vi "Laser Measurement Tool.vi"() -> ()   [LabVIEW 2017]
uses:
  Subsystems/Measurement/Typedefs/Measurement.Type--Enum.ctl
  Subsystems/Measurement/Typedefs/Configuration.SMU--Cluster.ctl
  Subsystems/SMU/Typedefs/Configuration--Cluster.ctl
  Subsystems/Measurement/Typedefs/Configuration.LIA--Cluster.ctl
  Subsystems/LIA/Typedefs/Configuration--Cluster.ctl
  Subsystems/Measurement/Typedefs/Configuration.OPM--Cluster.ctl
  Subsystems/OPM/Typedefs/Configuration--Cluster.ctl
  Subsystems/Measurement/Typedefs/Configuration.OPA--Cluster.ctl
  Subsystems/OPA/Typedefs/Configuration--Cluster.ctl
  Subsystems/Measurement.WavelengthSweeping/Typedefs/Configuration.Measurement--Cluster.ctl
  Subsystems/Measurement.Free/Measurement.Free.lvclass
  D:/upwork/Laser Measurement Tool/Laser/project/Subsystems/Measurement/Measurement.lvclass
  Subsystems/Measurement.Free.UI/Measurement.Free.UI.lvclass
  D:/upwork/Laser Measurement Tool/Laser/project/Subsystems/Measurement.UI/Measurement.UI.lvclass
  Subsystems/Measurement.WavelengthSweeping/Measurement.WavelengthSweeping.lvclass
  Subsystems/Measurement.WavelengthSweeping.UI/Measurement.WavelengthSweeping.UI.lvclass
  Subsystems/Measurement.Free/Typedefs/Configuration--Cluster.ctl
  Subsystems/Measurement.Free/Typedefs/Configuration.Hardware--Cluster.ctl
  Subsystems/Measurement.WavelengthSweeping/Typedefs/Configuration--Cluster.ctl
  Subsystems/Measurement.WavelengthSweeping/Typedefs/Configuration.Hardware--Cluster.ctl
  Subsystems/Measurement/Measurement.lvclass
  Subsystems/OPA.OrpheusHP/OPA.OrpheusHP.lvclass
  Subsystems/OPM.ThorlabsPM400/OPM.ThorlabsPM400.lvclass
  Subsystems/SMU/SMU.lvclass
  Subsystems/OPA/OPA.lvclass
  Subsystems/OPM/OPM.lvclass
  Subsystems/LIA/LIA.lvclass
panel:
  in  "OK":bool
  out "Measurements Tree":string(tree) caption="Chart A"
  in  "Add":bool
  in  "Remove":bool
  in  "Stop":bool
  in  "Start":bool
  in  "Measurement Parameters":T1(tab)
  in  "Delay time, ms":u16=500 step=100
  in  "Accumulation":u16=5 step=1
  in  "Integration time, s":dbl=5.0 step=0.1
  in  "OPA number of points":u16 step=1
  in  "OPA scan resolution, nm":dbl=20.0 step=10.0 format="%#_6f"
  in  "OPA stop wavelength, nm":dbl=1000.0 step=20.0 format="%#_6f"
  in  "OPA start wavelength, nm":dbl=600.0 step=20.0 format="%#_6f"
  in  "SMU voltage, V":dbl=1.0 step=0.01 format="%#_6f"
  in  "Sync":bool
  in  "Save":bool
  in  "Hardware Parameters":enum32{"Free"}(tab)
  in  "OPA Refresh List":bool
  in  "OPA Serial Number":string(combo)
  in  "OPM Refresh List":bool
  in  "OPM Simulated":bool
  in  "OPM Resource Name":string(combo)
  in  "SMU Channel":string(combo)="A"
  in  "SMU Simulated":bool
  in  "SMU VISA Resource Name":refnum<visa-resource-name>="GPIB0::26::INSTR"
  in  "LIA Simulated":bool
  in  "LIA VISA Resource Name":refnum<visa-resource-name>="GPIB0::8::INSTR"
  in  "Close":bool
  out "Status":string
  out "Progress":u8(slide) scale=0.0..100.0
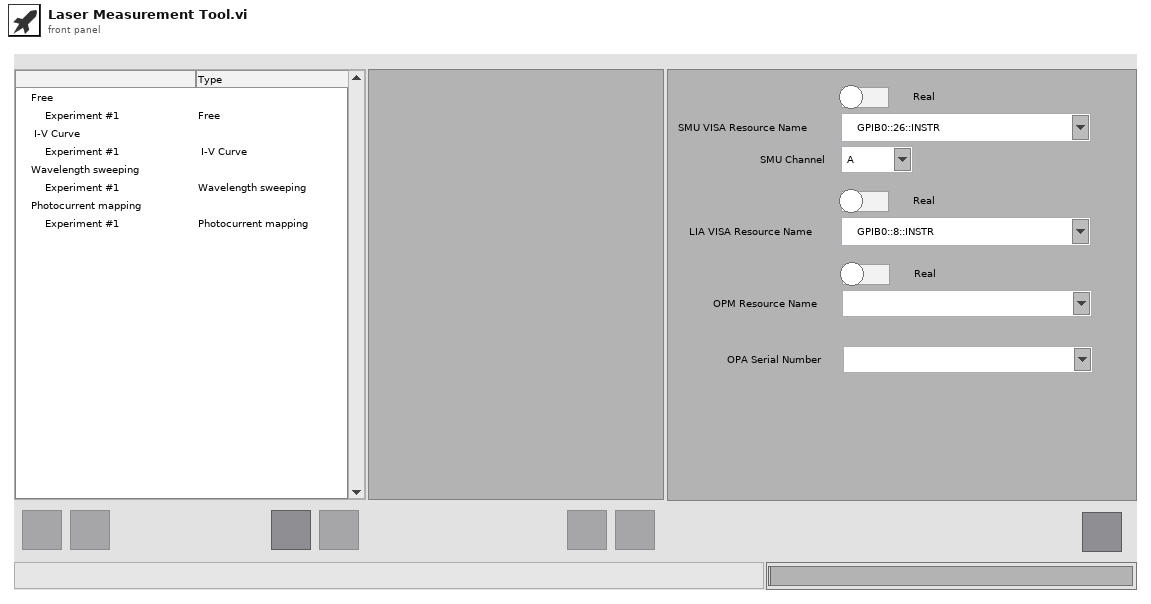
[diagram p1: front panel]
types:
  T1 = enum32{"Free", "I-V Curve", "Wavelength Sweeping", "Photocurrent mapping"}
  T2 = enum8{"Enabled", "Disabled", "Disabled and Grayed Out"}
  T3 = enum32{"Invalid", "Standard", "Closed", "Hidden", "Minimized", "Maximized"}
  T4 = enum32{"invalid app kind", "Development System", "Run Time System", "Student Edition", "Embedded LabVIEW", "Evaluation", "Custom"}
  T5 = typedef "Measurement.lvclass/Measurement.Type--Enum.ctl" = enum16{"Free", "I/V Curve", "Wavelength sweeping", "Photocurrent mapping"}
  T6 = typedef "LVPoint32TypeDef.ctl" = cluster{"Horizontal":i32, "Vertical":i32}
  T7 = typedef "Measurement.lvclass/Configuration.SMU--Cluster.ctl" = cluster{"Enable":bool, "SMU Model":string, "Configuration":T8}
  T8 = typedef "SMU.lvclass/Configuration--Cluster.ctl" = cluster{"VISA Resource":string, "Channel":string}
  T9 = typedef "Measurement.lvclass/Configuration.LIA--Cluster.ctl" = cluster{"Enable":bool, "LIA Model":string, "Configuration":T10}
  T10 = typedef "LIA.lvclass/Configuration--Cluster.ctl" = cluster{"VISA Resource":string}
  T11 = typedef "Measurement.lvclass/Configuration.OPM--Cluster.ctl" = cluster{"Enable":bool, "OPM Model":string, "Configuration":T12}
  T12 = typedef "OPM.lvclass/Configuration--Cluster.ctl" = cluster{"VISA Resource":string}
  T13 = typedef "Measurement.lvclass/Configuration.OPA--Cluster.ctl" = cluster{"Enable":bool, "OPA Model":string, "Configuration":T14}
  T14 = typedef "OPA.lvclass/Configuration--Cluster.ctl" = cluster{"Serial Number":string}
  T15 = typedef "Measurement.WavelengthSweeping.lvclass/Configuration.Measurement--Cluster.ctl" = cluster{"SMU Voltage, V":dbl, "OPA Start wavelength, nm":dbl, "OPA Stop wavelength, nm":dbl, "OPA Scan resolution, nm":dbl, "OPA Number or points":u16, "Integration time, sec":dbl, "Delay time, ms":u16, "Accumulation":u16}
  T16 = cluster{"Core":cluster{"Current VI Reference":refnum<vi>, "Close Panel on Exit?":bool}, "Measurements Tree":refnum<vi>, "Measurement.Type":T5, "Configuration":variant, "Configuration.SMU":T7, "Configuration.LIA":T9, "Configuration.OPM":T11, "Configuration.OPA":T13, "Configuration.Measurement.W-Sweep":T15}
  T17 = cluster{"Current VI Reference":refnum<vi>, "Close Panel on Exit?":bool}
  T18 = typedef "Measurement.Free.lvclass/Configuration--Cluster.ctl" = cluster{"Measurement.Type":T5, "Hardware":T19}
  T19 = typedef "Measurement.Free.lvclass/Configuration.Hardware--Cluster.ctl" = cluster{"SMU":T7, "LIA":T9, "OPM":T11, "OPA":T13}
  T20 = typedef "Measurement.WavelengthSweeping.lvclass/Configuration--Cluster.ctl" = cluster{"Measurement.Type":T5, "Hardware":T21, "Measurement":T15}
  T21 = typedef "Measurement.WavelengthSweeping.lvclass/Configuration.Hardware--Cluster.ctl" = cluster{"SMU":T7, "LIA":T9, "OPM":T11, "OPA":T13}
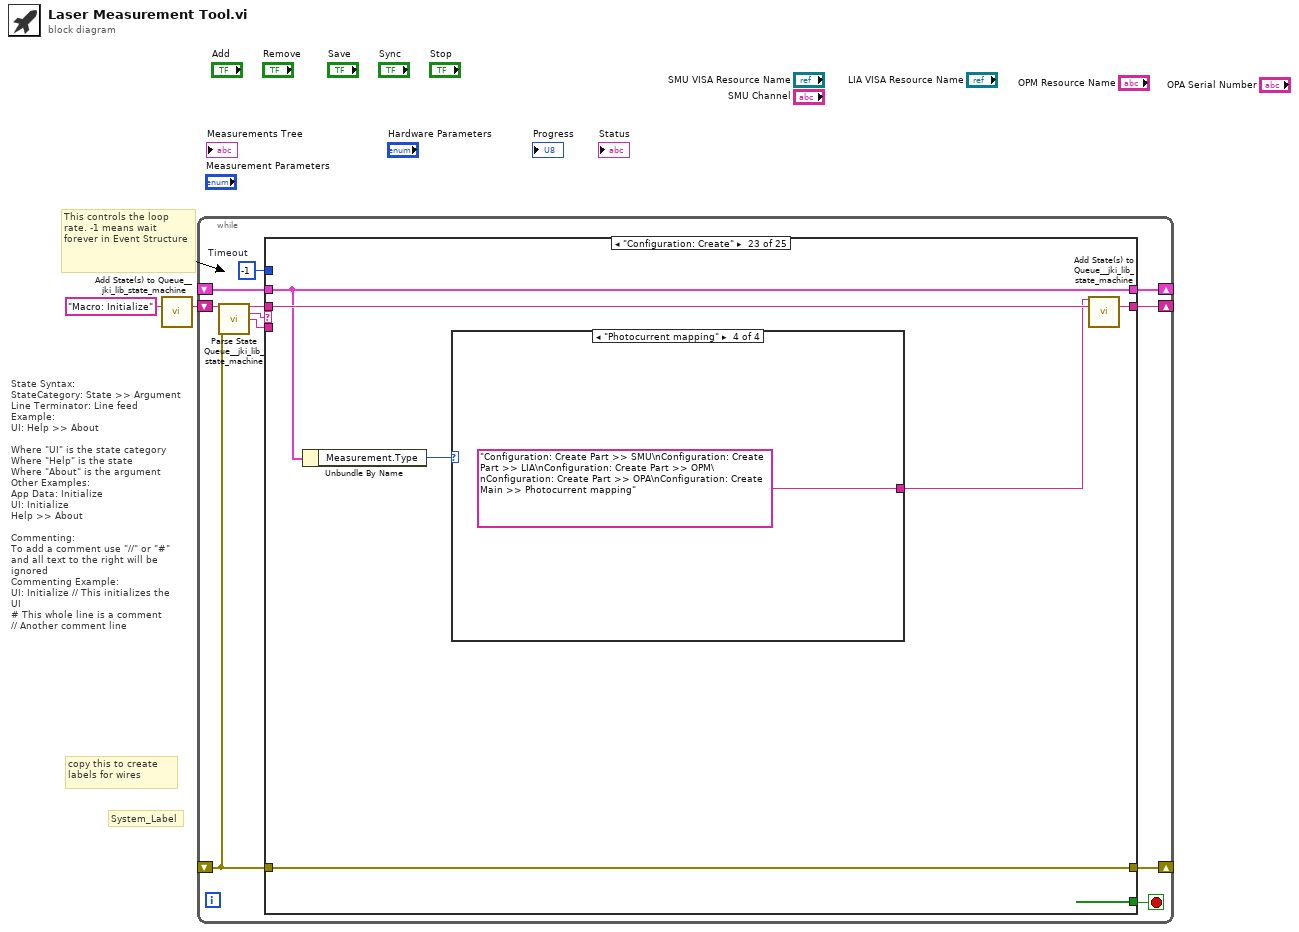
[diagram p0: block diagram]
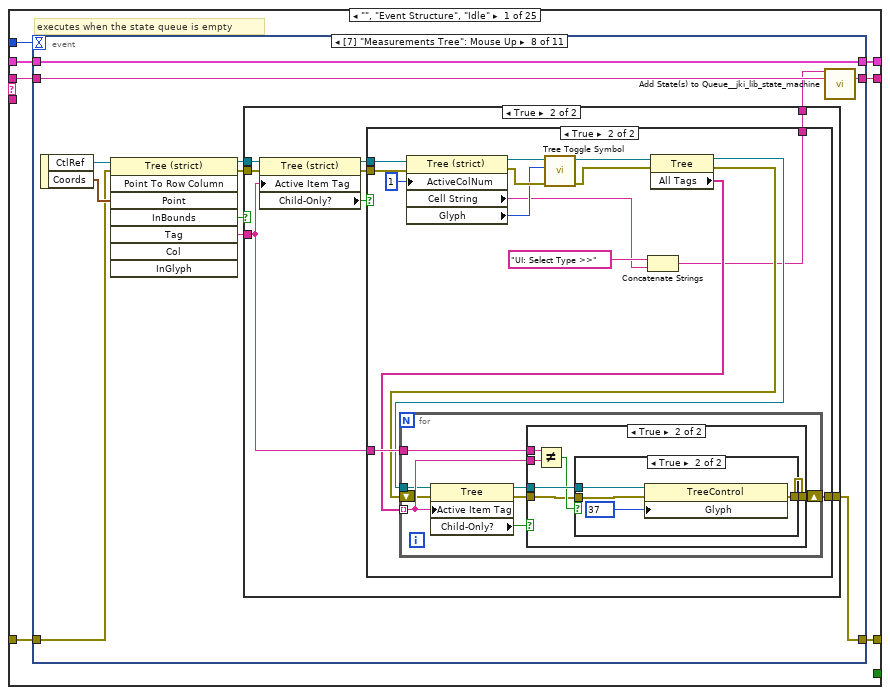
[diagram p2: hidden frame]
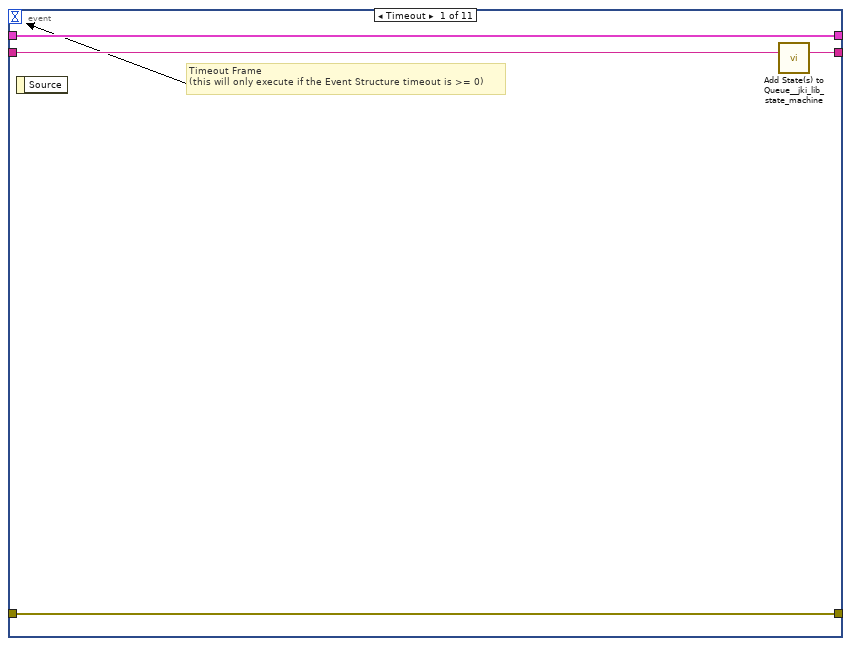
[diagram p3: hidden frame]
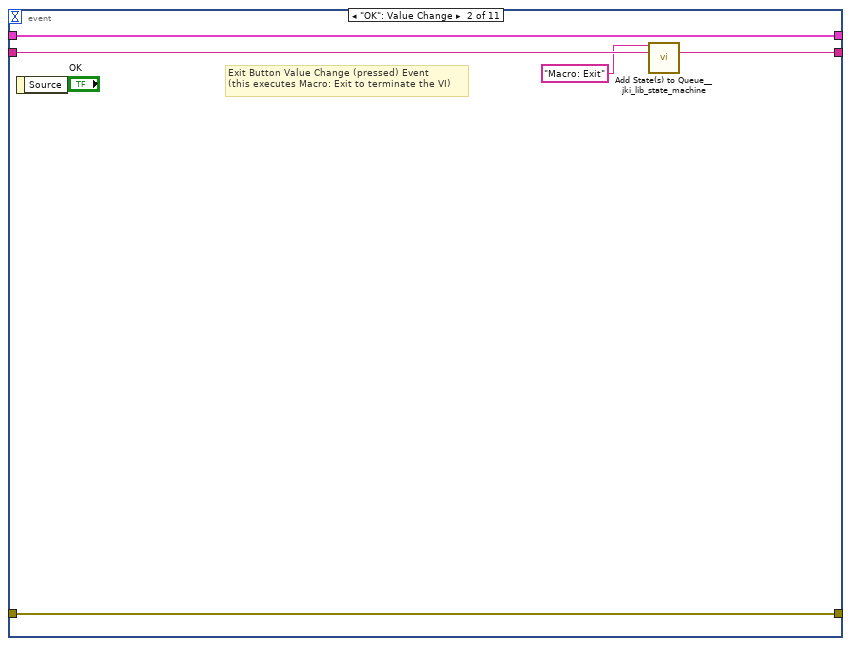
[diagram p4: hidden frame]
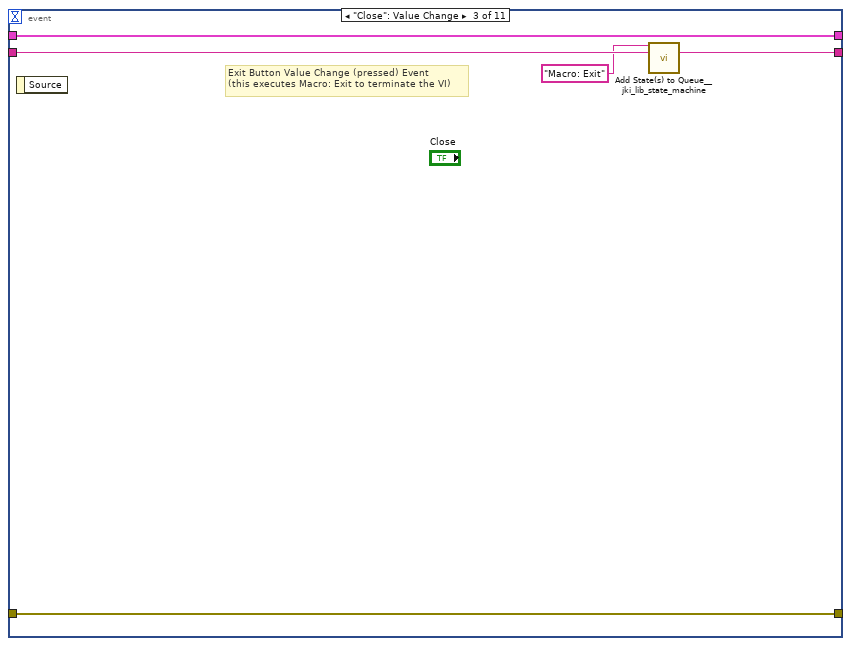
[diagram p5: hidden frame]
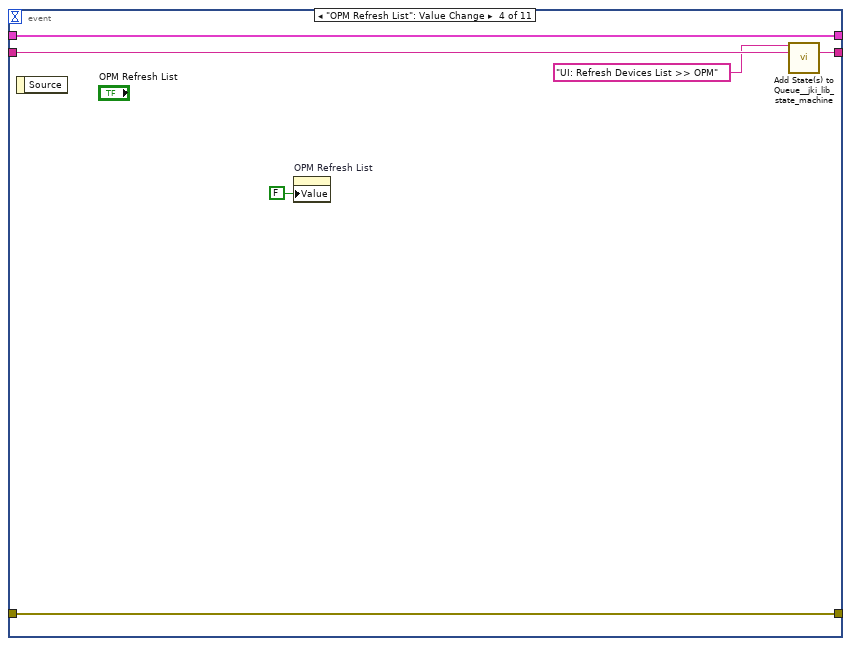
[diagram p6: hidden frame]
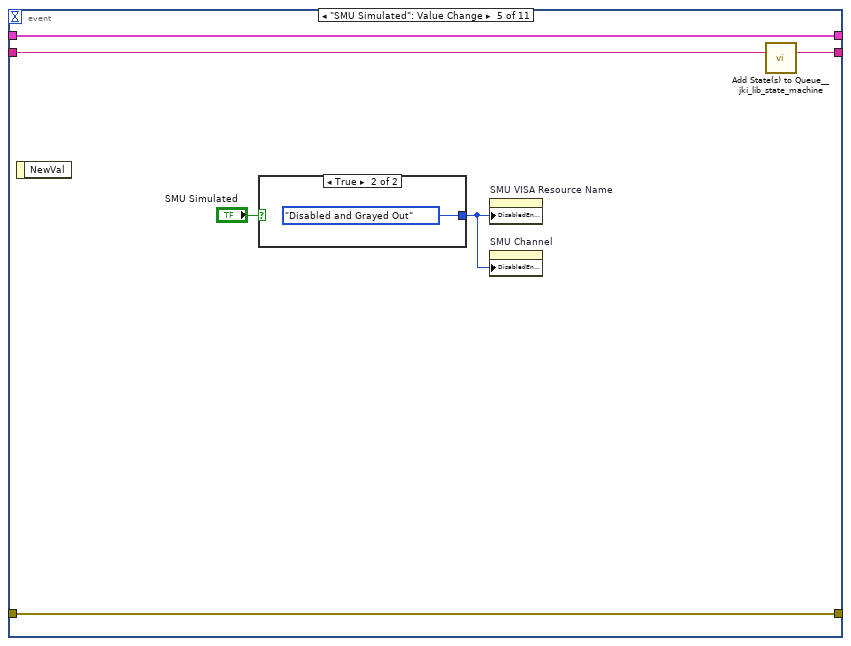
[diagram p7: hidden frame]
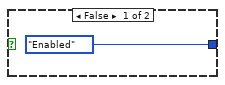
[diagram p8: hidden frame]
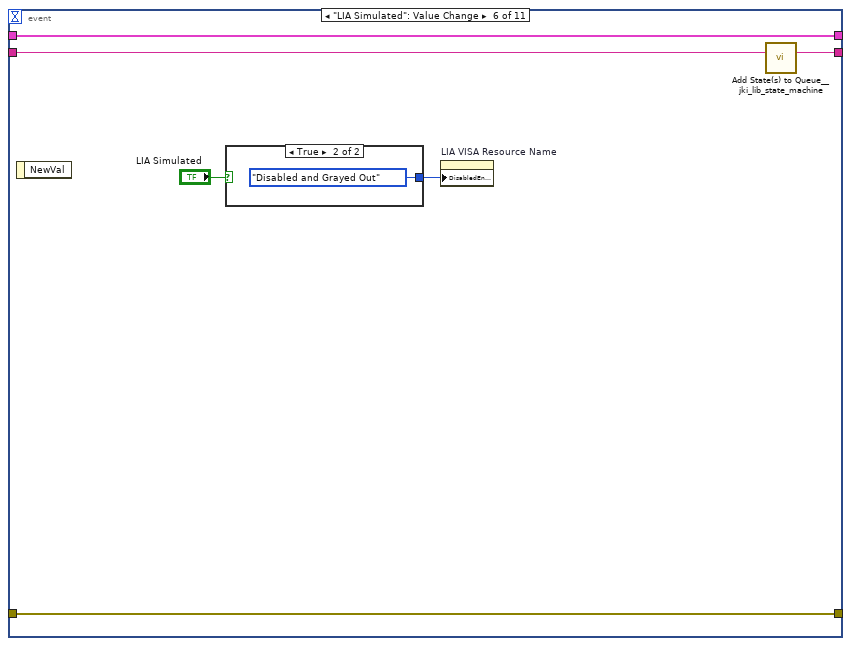
[diagram p9: hidden frame]
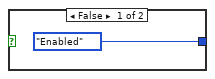
[diagram p10: hidden frame]
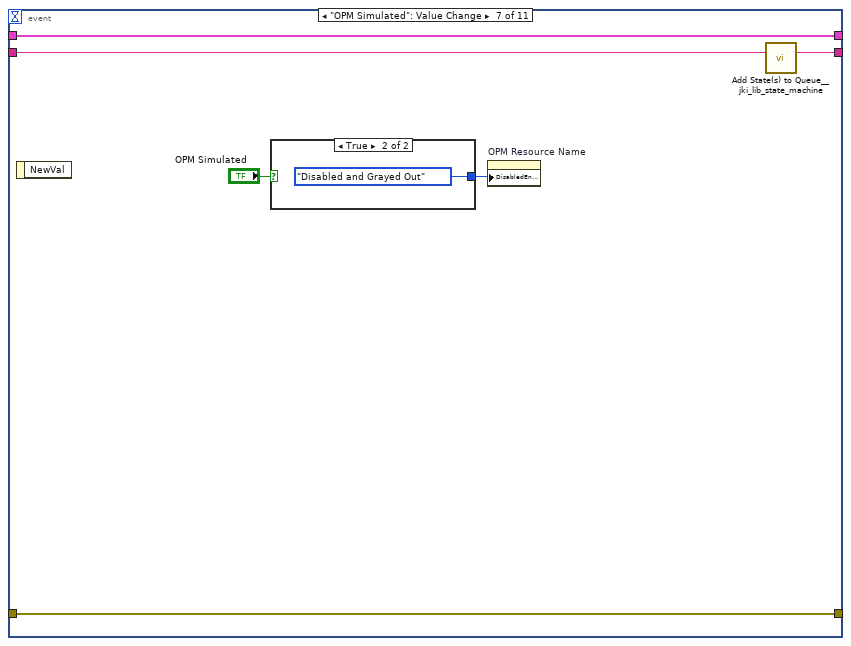
[diagram p11: hidden frame]
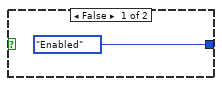
[diagram p12: hidden frame]
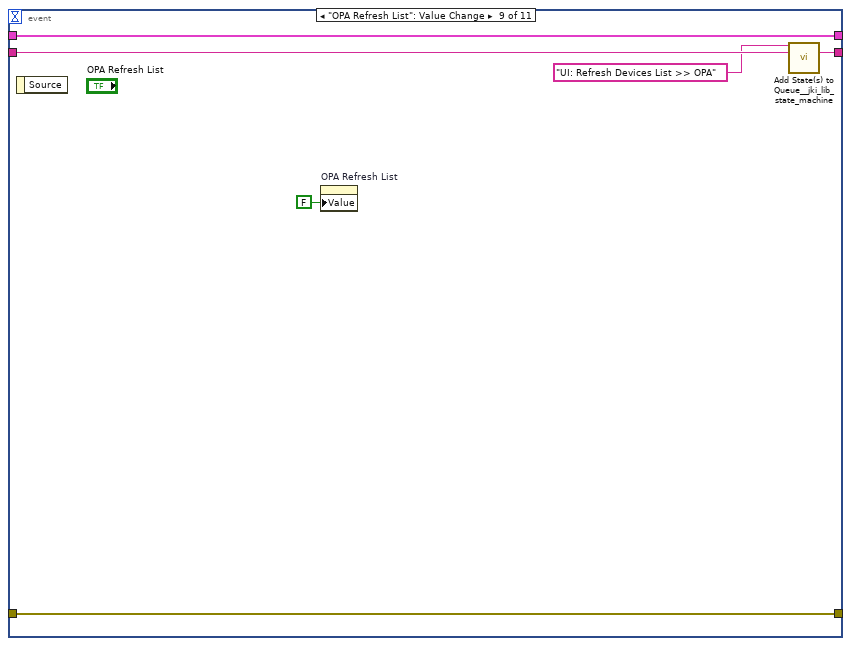
[diagram p17: hidden frame]
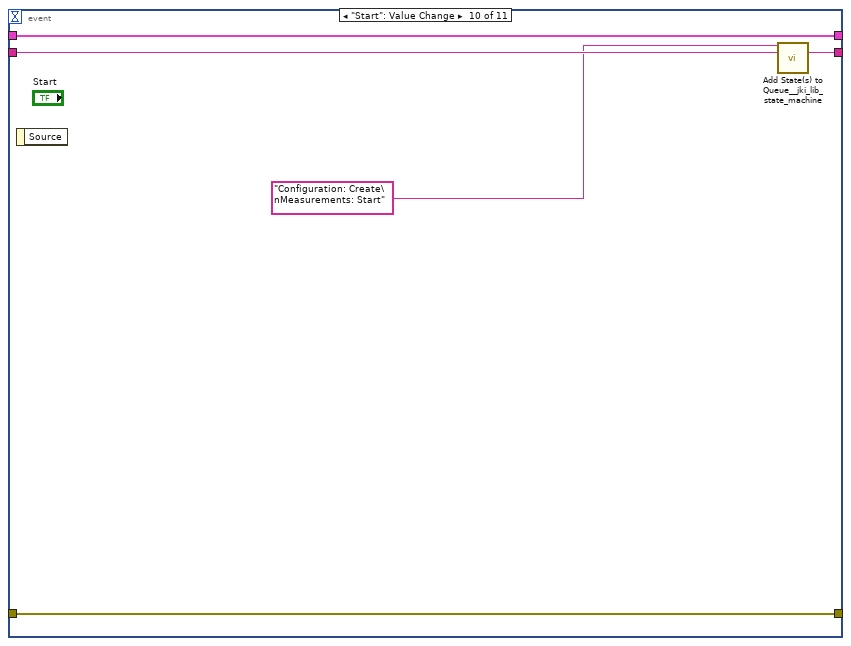
[diagram p18: hidden frame]
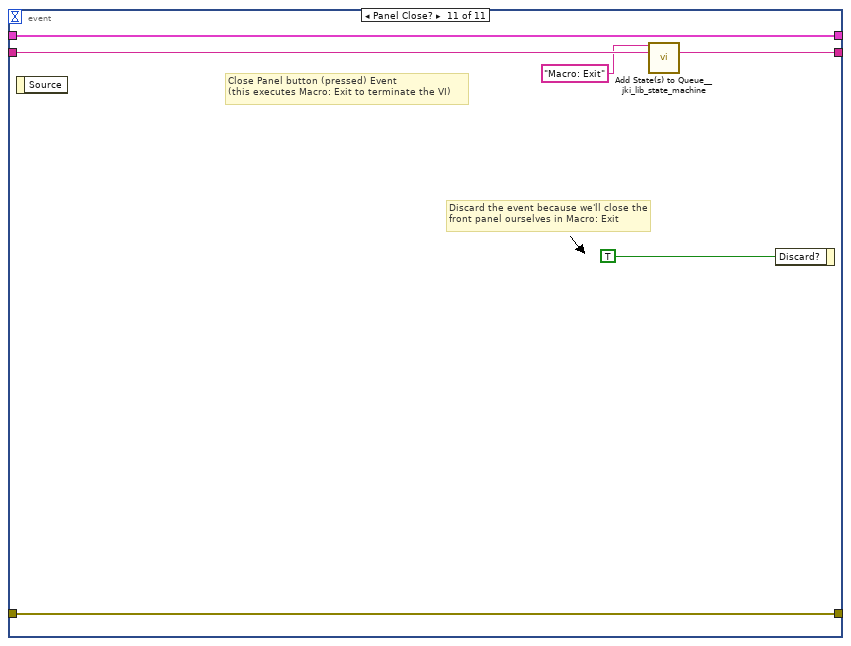
[diagram p19: hidden frame]
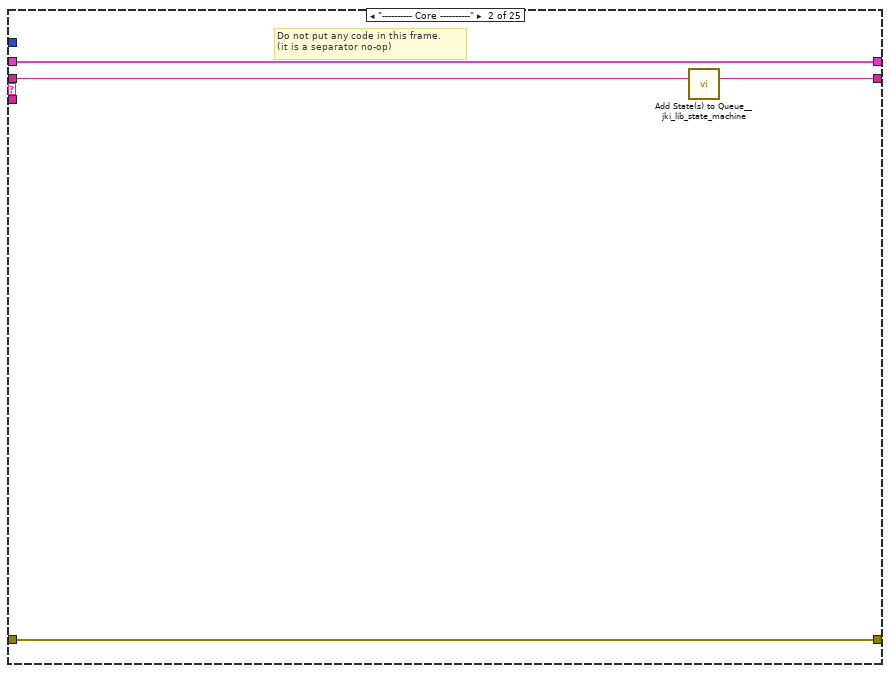
[diagram p20: hidden frame]
diagram:
  # "State Syntax:\nStateCategory: State >> Argument\nLine Terminator: Line feed\nExample:\nUI: Help >> About\n\nWhere \"UI\" is the state category\nWhere \"Help\" is the state\nWhere \"About\" is the argument\nOther Examples:\nApp Data: Initialize\nUI: Initialize\nHelp >> About\n\nCommenting:\nTo add a comment use \"//\" or \"#\" and all text to the right will be ignored\nCommenting Example:\nUI: Initialize // This initializes the UI\n# This whole line is a comment\n// Another comment line"
  # "copy this to create labels for wires"
  # "This controls the loop rate. -1 means wait forever in Event Structure"
  # "System_Label"
  n1 = call <vilib>:"Add State(s) to Queue__jki_lib_state_machine.vi"("State(s) in (\"\")"="Macro: Initialize") -> ("States Out"=w2:string)  [unwired: 14 in]
  n2 = while {
    shift-right: [w6] -> _
    shift-left: _ -> [w5]
    shift-right: [w9] -> _
    shift-left: _ -> [w3]
    shift-right: [w8] -> _
    shift-left: w2 -> [w10]
    stop <- w7 stop-if-true
    w4 = -1  # Timeout
    n3 = call <vilib>:"Parse State Queue__jki_lib_state_machine.vi"("State Queue"=w10, "Error In (no error)"=w3) -> ("Remaining States"=w12:string, "Current State"=w13:string, "Arguments"=w11:string)  [unwired: 11 in]
    n4 = case shown="\"Configuration: Create\"" w13 {
      selector: w13 -> [_ _ w144 _ _ _ _ _ _ _ _ _ _ _ _ _ _ _ _ _ _ _ _ _ _]
      tunnel: w12 -> [w20 w143 w148 w167 w173 w178 w182 w195 w201 w205 w210 w237 w260 w269 w282 w353 w377 w382 w392 w396 w405 w417 w423 w433 w489]
      tunnel: w11 -> [_ _ _ _ _ _ _ _ _ _ _ _ w255 w265 w276 w350 _ _ _ _ _ _ _ w430 w486]
      tunnel: w5 -> [w18 w140 w146 w160 w170 w176 w179 _ w196 w202 w208 w234 w258 w266 w278 w349 w374 w379 w389 w393 w403 w414 w420 w429 w485]
      tunnel: [w17 w141 w150 w164 errorcluster {"status"=FALSE, "code"=0, "source"=""} ("error out") w175 w180 w192 w197 w203 w207 w216 w256 w267 w279 w351 w375 w380 w390 w394 w398 w415 w421 w431 w487] -> w9
      tunnel: w3 -> [w16 w141 w149 w164 w169 w175 w180 w192 w198 w203 w207 w221 w257 w267 w280 w351 w375 w380 w390 w394 w399 w415 w421 w431 w487]
      tunnel: [w19 w142 w147 w166 w172 w177 w181 w194 w200 w204 w209 w236 w259 w268 w281 w352 w376 w381 w391 w395 w404 w416 w422 w432 w488] -> w8
      tunnel: [_ _ _ _ _ TRUE _ _ _ _ _ _ _ _ _ _ _ _ _ _ _ _ _ _ _] -> w7
      tunnel: [w15 w140 w146 w165 w170 w176 w179 w193 w196 w202 w208 w234 w258 w266 w278 w348 w374 w379 w389 w393 w403 w414 w420 w428 w484] -> w6
      tunnel: w4 -> [w14 _ _ _ _ _ _ _ _ _ _ _ _ _ _ _ _ _ _ _ _ _ _ _ _]
      frame "", "Event Structure", "Idle" {
        # "executes when the state queue is empty"
        n5 = event shown="[7] \"Measurements Tree\": Mouse Up" {
          selector: _ -> [_ _ _ _ _ _ _ _ _ _ _]
          dyn-events: _ -> [_ _ _ _ _ _ _ _ _ _ _]
          timeout: w14 -> [_ _ _ _ _ _ _ _ _ _ _]
          tunnel: w20 -> [w24 w29 w34 w40 w42 w52 w60 w74 w128 w131 w139]
          tunnel: [w23 w28 w33 w39 w43 w53 w61 w75 w127 w132 w138] -> w19
          tunnel: w18 -> [w21 w26 w31 w37 w44 w54 w62 w76 w125 w133 w136]
          tunnel: [w22 w27 w32 w38 w41 w51 w59 w67 w126 w130 w137] -> w17
          tunnel: w16 -> [w22 w27 w32 w38 w41 w51 w59 w66 w126 w130 w137]
          tunnel: [w21 w26 w31 w37 w44 w54 w62 w76 w125 w133 w136] -> w15
          event Timeout {
            # "Timeout Frame\n(this will only execute if the Event Structure timeout is >= 0)"
            n6 = event-data() -> ()  [unwired: 1 in, 1 out]
            n7 = call <vilib>:"Add State(s) to Queue__jki_lib_state_machine.vi"("State(s) in (\"\")"=w24) -> ("States Out"=w23:string)  [unwired: 14 in]
          }
          event "OK": Value Change {
            # "Exit Button Value Change (pressed) Event\n(this executes Macro: Exit to terminate the VI)"
            n8 = event-data() -> ()  [unwired: 1 in, 1 out]
            n9 = call <vilib>:"Add State(s) to Queue__jki_lib_state_machine.vi"("State(s) in Front (\"\")"="Macro: Exit", "State(s) in (\"\")"=w29) -> ("States Out"=w28:string)  [unwired: 13 in]
          }
          event "Close": Value Change {
            # "Exit Button Value Change (pressed) Event\n(this executes Macro: Exit to terminate the VI)"
            n10 = event-data() -> ()  [unwired: 1 in, 1 out]
            n11 = call <vilib>:"Add State(s) to Queue__jki_lib_state_machine.vi"("State(s) in Front (\"\")"="Macro: Exit", "State(s) in (\"\")"=w34) -> ("States Out"=w33:string)  [unwired: 13 in]
          }
          event "OPM Refresh List": Value Change {
            n12 = event-data() -> ()  [unwired: 1 in, 1 out]
            n13 = property on="OPM Refresh List" class="Bool (strict)"("Value"=FALSE ("OPM Refresh List")) -> ()  [unwired: 2 in, 2 out]
            n14 = call <vilib>:"Add State(s) to Queue__jki_lib_state_machine.vi"("State(s) in Front (\"\")"="UI: Refresh Devices List >> OPM", "State(s) in (\"\")"=w40) -> ("States Out"=w39:string)  [unwired: 13 in]
          }
          event "SMU Simulated": Value Change {
            n15 = event-data() -> ()  [unwired: 1 in, 1 out]
            n16 = case shown="True" "SMU Simulated" {
              tunnel: [T2."Enabled" ("Disabled") T2."Disabled and Grayed Out" ("Disabled")] -> w46
              frame False {
              }
              frame True {
              }
            }
            n17 = property on="SMU VISA Resource Name" class="VISAName"("DisabledEnum"=w46) -> ()  [unwired: 2 in, 2 out]
            n18 = property on="SMU Channel" class="CmbBox"("DisabledEnum"=w46) -> ()  [unwired: 2 in, 2 out]
            n19 = call <vilib>:"Add State(s) to Queue__jki_lib_state_machine.vi"("State(s) in (\"\")"=w42) -> ("States Out"=w43:string)  [unwired: 14 in]
          }
          event "LIA Simulated": Value Change {
            n20 = event-data() -> ()  [unwired: 1 in, 1 out]
            n21 = case shown="True" "LIA Simulated" {
              tunnel: [T2."Enabled" ("Disabled") T2."Disabled and Grayed Out" ("Disabled")] -> w50
              frame False {
              }
              frame True {
              }
            }
            n22 = property on="LIA VISA Resource Name" class="VISAName"("DisabledEnum"=w50) -> ()  [unwired: 2 in, 2 out]
            n23 = call <vilib>:"Add State(s) to Queue__jki_lib_state_machine.vi"("State(s) in (\"\")"=w52) -> ("States Out"=w53:string)  [unwired: 14 in]
          }
          event "OPM Simulated": Value Change {
            n24 = event-data() -> ()  [unwired: 1 in, 1 out]
            n25 = case shown="True" "OPM Simulated" {
              tunnel: [T2."Enabled" ("Disabled") T2."Disabled and Grayed Out" ("Disabled")] -> w58
              frame False {
              }
              frame True {
              }
            }
            n26 = property on="OPM Resource Name" class="CmbBox"("DisabledEnum"=w58) -> ()  [unwired: 2 in, 2 out]
            n27 = call <vilib>:"Add State(s) to Queue__jki_lib_state_machine.vi"("State(s) in (\"\")"=w60) -> ("States Out"=w61:string)  [unwired: 14 in]
          }
          event "Measurements Tree": Mouse Up {
            n28 = event-data() -> ("CtlRef"=w73:refnum<vi>, "Coords"=w72:T6)  [unwired: 1 in]
            n29 = invoke class="Tree (strict)" method="Point To Row Column"(reference=w73, error in=w66, "Point"=w72) -> (reference out=w70:refnum<vi>, error out=w69:errorcluster, "InBounds"=w71:bool, "Tag"=w68:string)  [unwired: 5 in, 4 out]
            n30 = case shown="True" w71 {
              tunnel: w70 -> [_ w85]
              tunnel: w69 -> [w77 w84]
              tunnel: w68 -> [_ w80]
              tunnel: [w77 w79] -> w67
              tunnel: [_ w78] -> w65
              frame False {
              }
              frame True {
                n31 = property class="Tree (strict)"(reference=w85, error in=w84, "Active Item Tag"=w80) -> (reference out=w82:refnum<vi>, error out=w81:errorcluster, "Child-Only?"=w83:bool)
                n32 = case shown="True" w83 {
                  tunnel: w82 -> [_ w101]
                  tunnel: w81 -> [w86 w102]
                  tunnel: w80 -> [_ w94]
                  tunnel: [w86 w88] -> w79
                  tunnel: [_ w87] -> w78
                  frame False {
                  }
                  frame True {
                    n33 = property class="Tree (strict)"(reference=w101, error in=w102, "ActiveColNum"=1 ("Active Cell:Active Column Number")) -> (reference out=w99:refnum<vi>, error out=w98:errorcluster, "Cell String"=w95:string, "Glyph"=w97:i32)
                    n34 = call "Tree Toggle Symbol.vi"("error in (no error)"=w98, "Symbol"=w97, "TreeControl in"=w99) -> ("error out"=w92:errorcluster, "TreeControl out"=w93:refnum<vi>)  [unwired: 6 in, 1 out]
                    n35 = Concatenate Strings("UI: Select Type >>", w95) -> (w87:string)
                    n36 = property class="Tree"(reference=w93, error in=w92) -> (reference out=w91:refnum<vi>, error out=w90:errorcluster, "All Tags"=w89:string[])
                    n37 = for {
                      tunnel: w89 -> [w108] mode=indexing
                      tunnel: w94 -> [w109]
                      tunnel: w91 -> [w106]
                      shift-right: [w103] -> w88
                      shift-left: w90 -> [w105]
                      n38 = property class="Tree"(reference=w106, error in=w105, "Active Item Tag"=w108) -> (reference out=w107:refnum<vi>, error out=w104:errorcluster, "Child-Only?"=w110:bool)
                      n39 = case shown="True" w110 {
                        tunnel: w109 -> [_ w117]
                        tunnel: w108 -> [_ w116]
                        tunnel: w107 -> [_ w115]
                        tunnel: w104 -> [w111 w113]
                        tunnel: [w111 w112] -> w103
                        frame False {
                        }
                        frame True {
                          n40 = Not Equal?(x=w117, y=w116) -> (x != y?=w114:bool)
                          n41 = case shown="True" w114 {
                            tunnel: w115 -> [_ w122]
                            tunnel: w113 -> [w118 w120]
                            tunnel: [w118 w119] -> w112
                            frame False {
                            }
                            frame True {
                              n42 = property class="TreeControl"(reference=w122, error in=w120, "Glyph"=37) -> (error out=w119:errorcluster)  [unwired: 1 out]
                            }
                          }
                        }
                      }
                    }
                  }
                }
              }
            }
            n43 = call <vilib>:"Add State(s) to Queue__jki_lib_state_machine.vi"("State(s) in Front (\"\")"=w65, "State(s) in (\"\")"=w74) -> ("States Out"=w75:string)  [unwired: 13 in]
          }
          event "OPA Refresh List": Value Change {
            n44 = event-data() -> ()  [unwired: 1 in, 1 out]
            n45 = property on="OPA Refresh List" class="Bool (strict)"("Value"=FALSE ("OPA Refresh List")) -> ()  [unwired: 2 in, 2 out]
            n46 = call <vilib>:"Add State(s) to Queue__jki_lib_state_machine.vi"("State(s) in Front (\"\")"="UI: Refresh Devices List >> OPA", "State(s) in (\"\")"=w128) -> ("States Out"=w127:string)  [unwired: 13 in]
          }
          event "Start": Value Change {
            n47 = event-data() -> ()  [unwired: 1 in, 1 out]
            n48 = call <vilib>:"Add State(s) to Queue__jki_lib_state_machine.vi"("State(s) in Front (\"\")"="Configuration: Create\nMeasurements: Start" ("State(s) in Front (\"\")"), "State(s) in (\"\")"=w131) -> ("States Out"=w132:string)  [unwired: 13 in]
          }
          event Panel Close? {
            # "Discard the event because we'll close the front panel ourselves in Macro: Exit"
            # "Close Panel button (pressed) Event\n(this executes Macro: Exit to terminate the VI)"
            n49 = event-data() -> ()  [unwired: 1 in, 1 out]
            n50 = call <vilib>:"Add State(s) to Queue__jki_lib_state_machine.vi"("State(s) in Front (\"\")"="Macro: Exit", "State(s) in (\"\")"=w139) -> ("States Out"=w138:string)  [unwired: 13 in]
            n51 = event-data("Discard?"=TRUE) -> ()  [unwired: 1 in, 1 out]
          }
        }
      }
      frame "---------- Core ----------" {
        # "Do not put any code in this frame.\n(it is a separator no-op)"
        n52 = call <vilib>:"Add State(s) to Queue__jki_lib_state_machine.vi"("State(s) in (\"\")"=w143) -> ("States Out"=w142:string)  [unwired: 14 in]
      }
      frame Default {
        w153 = 42 items=["No error", "Argument error", "Memory is full", "Out of zone", "End of file", "File already open", "Generic file I/O error", "File not found", "File permission error", "Disk is full", "Duplicate path", "Too many files open", "System feature not enabled", "Resource file not found", "Cannot add resource", "Resource not found", "Image not found", "Image memory error", "Pen does not exist", "Config type invalid", "Config token not found", "Config parse error", "Config memory error", "Bad external code format", "Bad external code offset", "External code not present", "Null window", "Destroy window error", "Null menu", "Print aborted", "Bad print record", "Print driver error", "Windows error during printing", "Memory error during printing", "Print dialog error", "Generic print error", "Invalid device refnum", "Device not found", "Device parameter error", "Device unit error", "Cannot open device", "Device call aborted", "Generic error", "Cancelled by user", "Object ID too low", "Object ID too high", "Object not in heap", "Unknown heap", "Unknown object (invalid DefProc)", "Unknown object (DefProc not in table)", "Message out of range", "Invalid (null) method", "Unknown message", "Manager call not supported", "Bad address", "Network operation in progress", "Network operation timed out", "Connection is busy", "Network attribute not supported", "Network error", "Address in use", "System out of memory", "Connection aborted", "Connection refused", "Not connected", "Already connected", "Connection closed", "Initialization error (interapplication manager)", "Bad occurrence", "Wait on unbound occurrence handler", "Occurrence queue overflow", "Datalog type conflict", "Unused", "Unrecognized type (interapplication manager)", "Memory corrupt", "Failed to make temporary DLL", "Old CIN version", "Drag socket not found", "Failed to load drop-object", "Failed to register OLE object", "Failed to release OLE object", "Format specifier type mismatch", "Unknown format specifier", "Too few format specifiers", "Too many format specifiers", "Scan failed", "Newer CIN version", "Error converting to variant", "Runtime menu error", "Password tampered", "Variant attribute not found", "Incompatible variant data type", "Event data is not available", "Event Store is not present", "Occurrence is not found", "Event Queue is not created", "Event info is not available", "Refnum passed is NULL", "Error retrieving Class GUID", "Error retrieving CoClass GUID", "Error retrieving TypeLib GUID.", "Bad built application magic bytes.", "Specific driver is different from the specific driver associated with the Logical Name.", "There is no session opened to the class driver.", "Max Error", "MAX - Error with config objects", "MAX - Error loading configuration", "MAX - Group not supported"]
        # "Current State"
        # "Do not delete, rename, or modify this frame.\n(this is used to capture unhandled states and typos)"
        # "Handle mistyped state name (developer tool)"
        n53 = Format Into String(format string="Software Exception: Unhandled State \"%s\"." ("message"), error in=w149, w144) -> (resulting string=w152:string, error out=w151:errorcluster)  [unwired: 1 in]
        n54 = call <vilib>:"Error Cluster From Error Code.vi"("show call chain? (False)"=TRUE, "error in (no error)"=w151, "error message (\"\")"=w152, "error code (0)"=w153) -> ("error out"=w150:errorcluster)  [unwired: 5 in]
        n55 = call <vilib>:"Add State(s) to Queue__jki_lib_state_machine.vi"("State(s) in (\"\")"=w148) -> ("States Out"=w147:string)  [unwired: 14 in]
      }
      frame "Initialize Core Data" {
        # "Do not delete, rename, or modify this frame.\n(this is used to determine panel behavior on exit)"
        # "originally closed?"
        # "exe?"
        # "If panel starts closed or is an EXE, then close it when we exit"
        n56 = property class="VI"() -> ("FP.State"=w157:T3)  [unwired: 2 in, 2 out]
        n57 = property class="App"() -> ("App.Kind"=w163:T4)  [unwired: 2 in, 2 out]
        n58 = control-ref of="Current VI Reference"() -> (w158:refnum<vi>)
        n59 = Equal?(x=w157, y=T3."Closed" ("Front Panel Window:State")) -> (x = y?=w155:bool)
        n60 = Equal?(x=w163, y=T4."Run Time System" ("Application:Kind")) -> (x = y?=w161:bool)
        n61 = Or(x=w155, y=w161) -> (x .or. y?=w159:bool)
        n62 = Bundle By Name(cluster=w160, "Core.Current VI Reference"=w158, "Core.Close Panel on Exit?"=w159) -> (w165:T16)
        n63 = call <vilib>:"Add State(s) to Queue__jki_lib_state_machine.vi"("State(s) in (\"\")"=w167) -> ("States Out"=w166:string)  [unwired: 14 in]
      }
      frame "Error Handler" {
        # "Unhandled Error -- Display it"
        # "Handle any errors here.\nYou can also output any states to clean-up after errors occur"
        # "Clear error"
        n64 = call <vilib>:"General Error Handler.vi"("error in (no error)"=w169) -> ()  [unwired: 10 in, 5 out]
        n65 = call <vilib>:"Add State(s) to Queue__jki_lib_state_machine.vi"("State(s) in Front (\"\")"="/* Post Error States", "State(s) in (\"\")"=w173) -> ("States Out"=w172:string)  [unwired: 13 in]
      }
      frame "Exit" {
        # "Do not put any code in this frame.\n(No errors that occur here will be handled.)"
        n66 = call <vilib>:"Add State(s) to Queue__jki_lib_state_machine.vi"("State(s) in (\"\")"=w178) -> ("States Out"=w177:string)  [unwired: 14 in]
      }
      frame "---------- Data ----------" {
        # "Do not put any code in this frame.\n(It is a separator no-op. You can make a copy of this frame to create a new Data frame)"
        n67 = call <vilib>:"Add State(s) to Queue__jki_lib_state_machine.vi"("State(s) in (\"\")"=w182) -> ("States Out"=w181:string)  [unwired: 14 in]
      }
      frame "Data: Initialize" {
        w183 = T15 {"SMU Voltage, V"=0.0, "OPA Start wavelength, nm"=0.0, "OPA Stop wavelength, nm"=0.0, "OPA Scan resolution, nm"=0.0, "OPA Number or points"=0, "Integration time, sec"=0.0, "Delay time, ms"=0, "Accumulation"=0}  # Configuration.Measurement.W-Sweep
        w184 = T13 {"Enable"=FALSE, "OPA Model"="", "Configuration"={"Serial Number"=""}}  # Configuration.OPA
        w185 = T11 {"Enable"=FALSE, "OPM Model"="", "Configuration"={"VISA Resource"=""}}  # Configuration.OPM
        w186 = T9 {"Enable"=FALSE, "LIA Model"="", "Configuration"={"VISA Resource"=""}}  # Configuration.LIA
        w187 = T7 {"Enable"=FALSE, "SMU Model"="", "Configuration"={"VISA Resource"="", "Channel"=""}}  # Configuration.SMU
        w188 = variant  # Configuration
        w189 = Measurement.Type--Enum."Free"  # Measurement.Type
        w191 = T17 {"Current VI Reference"=refnum, "Close Panel on Exit?"=FALSE}  # Core
        # "do not delete - used by framework"
        # "Data names and types of shift register data are defined by this bundle."
        # "Initialize the shift-register data, here.\n(data names are defined by what you wire into the bundle function)"
        n68 = control-ref of="Measurements Tree"() -> (w190:refnum<vi>)
        n69 = Bundle("Core"=w191, "Measurements Tree"=w190, "Measurement.Type"=w189, "Configuration"=w188, "Configuration.SMU"=w187, "Configuration.LIA"=w186, "Configuration.OPM"=w185, "Configuration.OPA"=w184, "Configuration.Measurement.W-Sweep"=w183) -> (w193:T16)  [unwired: 1 in]
        n70 = call <vilib>:"Add State(s) to Queue__jki_lib_state_machine.vi"("State(s) in (\"\")"=w195) -> ("States Out"=w194:string)  [unwired: 14 in]
      }
      frame "Data: Cleanup" {
        # "Cleanup any data and references, here.\n(this is called automatically, by the Macro: Exit)"
        n71 = Unbundle By Name(w196) -> ("Core.Current VI Reference"=w199:refnum<vi>)
        n72 = Close Reference(reference=w199, error in (no error)=w198) -> (error out=w197:errorcluster)
        n73 = call <vilib>:"Add State(s) to Queue__jki_lib_state_machine.vi"("State(s) in (\"\")"=w201) -> ("States Out"=w200:string)  [unwired: 14 in]
      }
      frame "---------- UI ----------" {
        # "Do not put any code in this frame.\n(It is a separator no-op. You can make a copy of this frame to create a new UI frame)"
        n74 = call <vilib>:"Add State(s) to Queue__jki_lib_state_machine.vi"("State(s) in (\"\")"=w205) -> ("States Out"=w204:string)  [unwired: 14 in]
      }
      frame "UI: Initialize" {
        # "Initialize the User Interface, here.\n(this is called automatically, by the Macro: Init)"
        n75 = call <vilib>:"Add State(s) to Queue__jki_lib_state_machine.vi"("State(s) in Front (\"\")"="UI: Tree Init\nUI: Refresh Devices List >> OPM\nUI: Refresh Devices List >> OPA\nUI: Select Type >> Free", "State(s) in (\"\")"=w210) -> ("States Out"=w209:string)  [unwired: 13 in]
      }
      frame "UI: Tree Init" {
        # "...add new measurement here..."
        # "Select Free mode \nas default"
        n76 = Unbundle By Name(w234) -> ("Measurements Tree"=w232:refnum<vi>)
        n77 = call <instrlib>:"Tree Empty.vi"("Tree Reference In"=w232, "error in (no error)"=w221) -> ("Tree Reference Out"=w235:refnum<vi>, "error out"=w230:errorcluster)  [unwired: 15 in, 1 out]
        n78 = call "Tree Create Measurement Item.vi"("error in (no error)"=w230, "New Text Value"="Free", "TreeControl in"=w235) -> ("error out"=w229:errorcluster, "Created Tag"=w218:string, "TreeControl out"=w231:refnum<vi>)  [unwired: 6 in]
        n79 = call "Tree Create Measurement Item.vi"("error in (no error)"=w229, "New Text Value"=" I-V Curve", "TreeControl in"=w231) -> ("error out"=w225:errorcluster, "TreeControl out"=w226:refnum<vi>)  [unwired: 6 in, 1 out]
        n80 = call "Tree Create Measurement Item.vi"("error in (no error)"=w225, "New Text Value"="Wavelength sweeping", "TreeControl in"=w226) -> ("error out"=w214:errorcluster, "TreeControl out"=w215:refnum<vi>)  [unwired: 6 in, 1 out]
        n81 = call "Tree Create Measurement Item.vi"("error in (no error)"=w214, "New Text Value"="Photocurrent mapping", "TreeControl in"=w215) -> ("error out"=w212:errorcluster, "TreeControl out"=w211:refnum<vi>)  [unwired: 6 in, 1 out]
        n82 = property on="Property Node" class="Tree"(reference=w211, error in=w212) -> (reference out=w224:refnum<vi>, error out=w222:errorcluster, "All Tags"=w223:string[])
        n83 = for {
          tunnel: w223 -> [w242] mode=indexing
          tunnel: w224 -> [w245]
          tunnel: [w241] -> w217
          shift-right: [w238] -> w219
          shift-left: w222 -> [w240]
          n84 = property class="Tree"(reference=w245, error in=w240, "Active Item Tag"=w242) -> (reference out=w244:refnum<vi>, error out=w239:errorcluster, "Child-Only?"=w243:bool)
          n85 = case shown="True" w243 {
            tunnel: w244 -> [w247 w252]
            tunnel: w242 -> [_ w251]
            tunnel: [w247 w250] -> w241
            tunnel: w239 -> [w246 w249]
            tunnel: [w246 w248] -> w238
            frame False {
            }
            frame True {
              n86 = property class="Tree"(reference=w252, error in=w249, "Active Item Tag"=w251, "Glyph"=37, "SelColor"=u32 16777216) -> (reference out=w250:refnum<vi>, error out=w248:errorcluster)
            }
          }
        }
        n87 = property class="Tree"(reference=w217, error in=w219, "Active Item Tag"=w218, "Glyph"=38) -> (error out=w216:errorcluster)  [unwired: 1 out]
        n88 = call <vilib>:"Add State(s) to Queue__jki_lib_state_machine.vi"("State(s) in (\"\")"=w237) -> ("States Out"=w236:string)  [unwired: 14 in]
      }
      frame "UI: Cursor Set" {
        # "Argument"
        # "Set and Unset Cursor Busy.\n(Usage: \"UI: Cursor Set >> Busy|Idle\")"
        n89 = case shown="\"Idle\", Default" w255 {
          tunnel: w257 -> [w262 w264]
          tunnel: [w261 w263] -> w256
          frame "Idle", Default {
            n90 = call <vilib>:"Unset Busy.vi"("error in (no error)"=w262) -> ("error out"=w261:errorcluster)  [unwired: 10 in]
          }
          frame "Busy" {
            n91 = call <vilib>:"Set Busy.vi"("error in (no error)"=w264) -> ("error out"=w263:errorcluster)  [unwired: 9 in, 1 out]
          }
        }
        n92 = call <vilib>:"Add State(s) to Queue__jki_lib_state_machine.vi"("State(s) in (\"\")"=w260) -> ("States Out"=w259:string)  [unwired: 14 in]
      }
      frame "UI: Refresh Devices List" {
        n93 = case shown="\"OPA\", Default" w265 {
          frame "OPA", Default {
            n94 = invoke on="OPA Serial Number" class="CmbBox" method="Reinit To Default"() -> (error out=w270:errorcluster)  [unwired: 3 in, 2 out]
            n95 = call "Locate Devices.vi"() -> ("Serial Numbers"=w271:string[])  [unwired: 2 in, 1 out]
            n96 = property on="OPA Serial Number" class="CmbBox"(error in=w270, "Strings[]"=w271) -> ()  [unwired: 1 in, 2 out]
            n97 = Index Array(array=w271) -> (element=w272:string)  [unwired: 1 in]
            n98 = property on="OPA Serial Number" class="CmbBox"("Value"=w272) -> ()  [unwired: 2 in, 2 out]
          }
          frame "OPM" {
            n99 = invoke on="OPM Resource Name" class="CmbBox" method="Reinit To Default"() -> (error out=w273:errorcluster)  [unwired: 3 in, 2 out]
            n100 = call "Find Resources.vi"() -> ("Resource Names"=w274:string[])  [unwired: 2 in, 1 out]
            n101 = property on="OPM Resource Name" class="CmbBox"(error in=w273, "Strings[]"=w274) -> ()  [unwired: 1 in, 2 out]
            n102 = Index Array(array=w274) -> (element=w275:string)  [unwired: 1 in]
            n103 = property on="OPM Resource Name" class="CmbBox"("Value"=w275) -> ()  [unwired: 2 in, 2 out]
          }
        }
        n104 = call <vilib>:"Add State(s) to Queue__jki_lib_state_machine.vi"("State(s) in (\"\")"=w269) -> ("States Out"=w268:string)  [unwired: 14 in]
      }
      frame "UI: Front Panel State" {
        # "Argument"
        # "Set Front Panel Open or Closed\n(Usage: \"UI: Front Panel State >> Open|Close\")"
        n105 = Unbundle By Name(w278) -> ("Core.Current VI Reference"=w277:refnum<vi>)
        n106 = case shown="\"Minimize\", \"Minimized\"" w276 {
          tunnel: w280 -> [w288 w303 w314 w327 w340]
          tunnel: [w290 w304 w316 w329 w342] -> w279
          tunnel: w277 -> [w289 w301 w315 w328 w341]
          frame "Open", "Standard", Default {
            w283 = T3."Standard" ("State")
            n107 = property class="VI"(reference=w289, error in=w288) -> (reference out=w286:refnum<vi>, error out=w287:errorcluster, "FP.State"=w285:T3)
            n108 = Not Equal?(x=w285, y=w283) -> (x != y?=w284:bool)
            n109 = case shown="True" w284 {
              tunnel: [w294 w296] -> w290
              tunnel: w287 -> [w293 w296]
              tunnel: w286 -> [w292 _]
              tunnel: w283 -> [w291 _]
              frame True {
                n110 = invoke class="VI" method="FP.Open"(reference=w292, error in=w293, "Activate"=TRUE, "State"=w291) -> (error out=w294:errorcluster)  [unwired: 1 in, 4 out]
              }
              frame False {
              }
            }
          }
          frame "Close", "Closed" {
            n111 = property class="VI"(reference=w301, error in=w303) -> (reference out=w300:refnum<vi>, error out=w302:errorcluster, "FP.State"=w298:T3)
            n112 = Not Equal?(x=w298, y=T3."Closed" ("Front Panel Window:State")) -> (x != y?=w297:bool)
            n113 = case shown="True" w297 {
              tunnel: [w305 w308] -> w304
              tunnel: w302 -> [w305 w307]
              tunnel: w300 -> [_ w306]
              frame False {
              }
              frame True {
                n114 = invoke class="VI" method="FP.Close"(reference=w306, error in=w307) -> (error out=w308:errorcluster)  [unwired: 1 in, 2 out]
              }
            }
          }
          frame "Hidden", "Hide" {
            w309 = T3."Hidden" ("State")
            n115 = property class="VI"(reference=w315, error in=w314) -> (reference out=w312:refnum<vi>, error out=w313:errorcluster, "FP.State"=w311:T3)
            n116 = Not Equal?(x=w311, y=w309) -> (x != y?=w310:bool)
            n117 = case shown="True" w310 {
              tunnel: [w320 w321] -> w316
              tunnel: w313 -> [w319 w321]
              tunnel: w312 -> [w318 _]
              tunnel: w309 -> [w317 _]
              frame True {
                n118 = invoke class="VI" method="FP.Open"(reference=w318, error in=w319, "State"=w317) -> (error out=w320:errorcluster)  [unwired: 2 in, 4 out]
              }
              frame False {
              }
            }
          }
          frame "Minimize", "Minimized" {
            w322 = T3."Minimized" ("State")
            n119 = property class="VI"(reference=w328, error in=w327) -> (reference out=w325:refnum<vi>, error out=w326:errorcluster, "FP.State"=w324:T3)
            n120 = Not Equal?(x=w324, y=w322) -> (x != y?=w323:bool)
            n121 = case shown="True" w323 {
              tunnel: [w333 w334] -> w329
              tunnel: w326 -> [w332 w334]
              tunnel: w325 -> [w331 _]
              tunnel: w322 -> [w330 _]
              frame True {
                n122 = invoke class="VI" method="FP.Open"(reference=w331, error in=w332, "State"=w330) -> (error out=w333:errorcluster)  [unwired: 2 in, 4 out]
              }
              frame False {
              }
            }
          }
          frame "Maximize", "Maximized" {
            w335 = T3."Maximized" ("State")
            n123 = property class="VI"(reference=w341, error in=w340) -> (reference out=w338:refnum<vi>, error out=w339:errorcluster, "FP.State"=w337:T3)
            n124 = Not Equal?(x=w337, y=w335) -> (x != y?=w336:bool)
            n125 = case shown="True" w336 {
              tunnel: [w346 w347] -> w342
              tunnel: w339 -> [w345 w347]
              tunnel: w338 -> [w344 _]
              tunnel: w335 -> [w343 _]
              frame True {
                n126 = invoke class="VI" method="FP.Open"(reference=w344, error in=w345, "State"=w343) -> (error out=w346:errorcluster)  [unwired: 2 in, 4 out]
              }
              frame False {
              }
            }
          }
        }
        n127 = call <vilib>:"Add State(s) to Queue__jki_lib_state_machine.vi"("State(s) in (\"\")"=w282) -> ("States Out"=w281:string)  [unwired: 14 in]
      }
      frame "UI: Select Type" {
        n128 = case shown="\"Free\", Default" w350 {
          tunnel: w349 -> [w358 w363 w366 w373]
          tunnel: [w356 w362 w367 w372] -> w348
          frame "Free", Default {
            n129 = Bundle By Name(cluster=w358, "Measurement.Type"=Measurement.Type--Enum."Free") -> (w356:T16)
            n130 = property on="Measurement Parameters" class="TabCtl (strict)"("Value"=T1."Free" ("Measurement Parameters")) -> ()  [unwired: 2 in, 2 out]
            n131 = property on="Status" class="Str"("Value"="Free measurement mode" ("Status")) -> ()  [unwired: 2 in, 2 out]
          }
          frame "I-V Curve" {
            n132 = Bundle By Name(cluster=w363, "Measurement.Type"=Measurement.Type--Enum."I/V Curve") -> (w362:T16)
            n133 = property on="Measurement Parameters" class="TabCtl (strict)"("Value"=T1."I-V Curve" ("Measurement Parameters")) -> ()  [unwired: 2 in, 2 out]
            n134 = property on="Status" class="Str"("Value"="I/V curve measurement mode" ("Status")) -> ()  [unwired: 2 in, 2 out]
          }
          frame "Wavelength sweeping" {
            n135 = Bundle By Name(cluster=w366, "Measurement.Type"=Measurement.Type--Enum."Wavelength sweeping") -> (w367:T16)
            n136 = property on="Measurement Parameters" class="TabCtl (strict)"("Value"=T1."Wavelength Sweeping" ("Measurement Parameters")) -> ()  [unwired: 2 in, 2 out]
            n137 = property on="Status" class="Str"("Value"=" Wavelength Sweeping measurement mode" ("Status")) -> ()  [unwired: 2 in, 2 out]
          }
          frame "Photocurrent mapping" {
            n138 = Bundle By Name(cluster=w373, "Measurement.Type"=Measurement.Type--Enum."Photocurrent mapping") -> (w372:T16)
            n139 = property on="Measurement Parameters" class="TabCtl (strict)"("Value"=T1."Photocurrent mapping" ("Measurement Parameters")) -> ()  [unwired: 2 in, 2 out]
            n140 = property on="Status" class="Str"("Value"=" Photocurrent mapping measurement mode" ("Status")) -> ()  [unwired: 2 in, 2 out]
          }
        }
        n141 = call <vilib>:"Add State(s) to Queue__jki_lib_state_machine.vi"("State(s) in (\"\")"=w353) -> ("States Out"=w352:string)  [unwired: 14 in]
      }
      frame "---------- Macro ----------" {
        # "Do not put any code in this frame.\n(It is a separator no-op. You can make a copy of this frame to create a new Macro frame)"
        n142 = call <vilib>:"Add State(s) to Queue__jki_lib_state_machine.vi"("State(s) in (\"\")"=w377) -> ("States Out"=w376:string)  [unwired: 14 in]
      }
      frame "Macro: Initialize" {
        # "Initialization Macro\n(This is called once, when the VI starts)"
        n143 = call <vilib>:"Add State(s) to Queue__jki_lib_state_machine.vi"("State(s) in Front (\"\")"="Data: Initialize\nInitialize Core Data\nUI: Initialize\nUI: Front Panel State >> Open", "State(s) in (\"\")"=w382) -> ("States Out"=w381:string)  [unwired: 13 in]
      }
      frame "Macro: Exit" {
        # "Exit Macro\n(This is called once, when the VI exits)"
        n144 = Unbundle By Name(w389) -> ("Core.Close Panel on Exit?"=w388:bool)
        n145 = Select(t="UI: Front Panel State >> Close", s=w388, f="") -> (s? t:f=w385:string)
        n146 = call <vilib>:"Add State(s) to Queue__jki_lib_state_machine.vi"("State(s) in (\"\")"=w385, "State(s) at Back (\"\")"="Data: Cleanup\nExit") -> ("States Out"=w383:string)  [unwired: 13 in]
        n147 = call <vilib>:"Add State(s) to Queue__jki_lib_state_machine.vi"("State(s) in Front (\"\")"=w383, "State(s) in (\"\")"=w392) -> ("States Out"=w391:string)  [unwired: 13 in]
      }
      frame "---------- Measurements ----------" {
        # "Template Separator\n(You can make a copy of, or modify, this frame)"
        n148 = call <vilib>:"Add State(s) to Queue__jki_lib_state_machine.vi"("State(s) in (\"\")"=w396) -> ("States Out"=w395:string)  [unwired: 14 in]
      }
      frame "Measurements: Start" {
        n149 = Unbundle By Name(w403) -> ("Measurement.Type"=w402:T5, "Configuration"=w397:variant)
        n150 = case shown="\"Free\", Default" w402 {
          tunnel: [w407 w409 w411 w413] -> w401
          tunnel: [w406 w408 w410 w412] -> w400
          frame "Free", Default {
            w406 = refnum<class "Measurement.Free.UI.lvclass"> refnum  # Measurement.Free.UI
            w407 = refnum<class "Measurement.Free.lvclass"> refnum  # Measurement.Free
          }
          frame "I/V Curve" {
            w408 = refnum<class "Measurement.Free.UI.lvclass"> refnum  # Measurement.Free.UI
            w409 = refnum<class "Measurement.Free.lvclass"> refnum  # Measurement.Free
          }
          frame "Wavelength sweeping" {
            w410 = refnum<class "Measurement.WavelengthSweeping.UI.lvclass"> refnum  # Measurement.WavelengthSweeping.UI
            w411 = refnum<class "Measurement.WavelengthSweeping.lvclass"> refnum  # Measurement.WavelengthSweeping
          }
          frame "Photocurrent mapping" {
            w412 = refnum<class "Measurement.Free.UI.lvclass"> refnum  # Measurement.Free.UI
            w413 = refnum<class "Measurement.Free.lvclass"> refnum  # Measurement.Free
          }
        }
        n151 = call "Measurement Launcher.vi"("error in (no error)"=w399, "Configuration"=w397, "Measurement.UI"=w400, "Measurement"=w401) -> ("error out"=w398:errorcluster)  [unwired: 7 in]
        n152 = call <vilib>:"Add State(s) to Queue__jki_lib_state_machine.vi"("State(s) in (\"\")"=w405) -> ("States Out"=w404:string)  [unwired: 14 in]
      }
      frame "---------- Configuration ----------" {
        # "Do not put any code in this frame.\n(it is a separator no-op)"
        n153 = call <vilib>:"Add State(s) to Queue__jki_lib_state_machine.vi"("State(s) in (\"\")"=w417) -> ("States Out"=w416:string)  [unwired: 14 in]
      }
      frame "Configuration: Create" {
        n154 = Unbundle By Name(w420) -> ("Measurement.Type"=w419:T5)
        n155 = case shown="\"Photocurrent mapping\"" w419 {
          tunnel: ["Configuration: Create Part >> SMU\nConfiguration: Create Part >> LIA\nConfiguration: Create Part >> OPM\nConfiguration: Create Part >> OPA\nConfiguration: Create Main >> Free" ("State(s) in Front (\"\")") "Configuration: Create Part >> SMU\nConfiguration: Create Part >> LIA\nConfiguration: Create Part >> OPM\nConfiguration: Create Part >> OPA\nConfiguration: Create Main >> I-V Curve" ("State(s) in Front (\"\")") "Configuration: Create Part >> SMU\nConfiguration: Create Part >> LIA\nConfiguration: Create Part >> OPM\nConfiguration: Create Part >> OPA\nConfiguration: Create Main >> Wavelength sweeping" ("State(s) in Front (\"\")") "Configuration: Create Part >> SMU\nConfiguration: Create Part >> LIA\nConfiguration: Create Part >> OPM\nConfiguration: Create Part >> OPA\nConfiguration: Create Main >> Photocurrent mapping" ("State(s) in Front (\"\")")] -> w418
          frame "Free", Default {
          }
          frame "I/V Curve" {
          }
          frame "Wavelength sweeping" {
          }
          frame "Photocurrent mapping" {
          }
        }
        n156 = call <vilib>:"Add State(s) to Queue__jki_lib_state_machine.vi"("State(s) in Front (\"\")"=w418, "State(s) in (\"\")"=w423) -> ("States Out"=w422:string)  [unwired: 13 in]
      }
      frame "Configuration: Create Part" {
        n157 = case shown="\"SMU\", Default" w430 {
          tunnel: w429 -> [w435 w447 w456 w467 w474]
          tunnel: [w434 w446 w457 w466 w473] -> w428
          frame "SMU", Default {
            w439 = T7 {"Enable"=FALSE, "SMU Model"="", "Configuration"={"VISA Resource"="", "Channel"=""}}  # Configuration.SMU
            n158 = property on="SMU Simulated" class="Bool (strict)"() -> ("Value"=w437:bool)  [unwired: 2 in, 2 out]
            n159 = case shown="False" w437 {
              tunnel: ["Keithley2600" ("SMU Model") "Simulated" ("SMU Model")] -> w438
              frame False {
              }
              frame True {
              }
            }
            n160 = property on="SMU VISA Resource Name" class="VISAName"() -> ("Value"=w441:refnum<visa-resource-name>)  [unwired: 2 in, 2 out]
            n161 = property on="SMU Channel" class="CmbBox"() -> ("Value"=w442:string)  [unwired: 2 in, 2 out]
            n162 = Bundle By Name(cluster=w439, "Enable"=TRUE, "SMU Model"=w438, "Configuration.VISA Resource"=w441, "Configuration.Channel"=w442) -> (w436:T7)
            n163 = Bundle By Name(cluster=w435, "Configuration.SMU"=w436) -> (w434:T16)
          }
          frame "LIA" {
            w449 = T9 {"Enable"=FALSE, "LIA Model"="", "Configuration"={"VISA Resource"=""}}  # Configuration.LIA
            n164 = property on="LIA Simulated" class="Bool (strict)"() -> ("Value"=w452:bool)  [unwired: 2 in, 2 out]
            n165 = case shown="False" w452 {
              tunnel: ["SR810" ("SMU Model") "Simulated" ("SMU Model")] -> w450
              frame False {
              }
              frame True {
              }
            }
            n166 = property on="LIA VISA Resource Name" class="VISAName"() -> ("Value"=w451:refnum<visa-resource-name>)  [unwired: 2 in, 2 out]
            n167 = Bundle By Name(cluster=w449, "Enable"=TRUE, "LIA Model"=w450, "Configuration.VISA Resource"=w451) -> (w445:T9)
            n168 = Bundle By Name(cluster=w447, "Configuration.LIA"=w445) -> (w446:T16)
          }
          frame "OPM" {
            w459 = T11 {"Enable"=FALSE, "OPM Model"="", "Configuration"={"VISA Resource"=""}}  # Configuration.OPM
            n169 = property on="OPM Simulated" class="Bool (strict)"() -> ("Value"=w462:bool)  [unwired: 2 in, 2 out]
            n170 = case shown="False" w462 {
              tunnel: ["ThorlabsPM400" ("SMU Model") "Simulated" ("SMU Model")] -> w460
              frame False {
              }
              frame True {
              }
            }
            n171 = property on="OPM Resource Name" class="CmbBox"() -> ("Value"=w461:string)  [unwired: 2 in, 2 out]
            n172 = Bundle By Name(cluster=w459, "Enable"=TRUE, "OPM Model"=w460, "Configuration.VISA Resource"=w461) -> (w455:T11)
            n173 = Bundle By Name(cluster=w456, "Configuration.OPM"=w455) -> (w457:T16)
          }
          frame "OPA" {
            w470 = T13 {"Enable"=FALSE, "OPA Model"="", "Configuration"={"Serial Number"=""}}  # Configuration.OPA
            n174 = property on="OPA Serial Number" class="CmbBox"() -> ("Value"=w471:string)  [unwired: 2 in, 2 out]
            n175 = Bundle By Name(cluster=w470, "Enable"=TRUE, "OPA Model"="OrpheusHP", "Configuration.Serial Number"=w471) -> (w465:T13)
            n176 = Bundle By Name(cluster=w467, "Configuration.OPA"=w465) -> (w466:T16)
          }
          frame "Wavelength sweeping" {
            w475 = T15 {"SMU Voltage, V"=0.0, "OPA Start wavelength, nm"=0.0, "OPA Stop wavelength, nm"=0.0, "OPA Scan resolution, nm"=0.0, "OPA Number or points"=0, "Integration time, sec"=0.0, "Delay time, ms"=0, "Accumulation"=0}  # Configuration.Measurement
            n177 = Bundle By Name(cluster=w475, "SMU Voltage, V"="SMU voltage, V", "OPA Start wavelength, nm"="OPA start wavelength, nm", "OPA Stop wavelength, nm"="OPA stop wavelength, nm", "OPA Scan resolution, nm"="OPA scan resolution, nm", "OPA Number or points"="OPA number of points", "Integration time, sec"="Integration time, s", "Delay time, ms"="Delay time, ms", "Accumulation"="Accumulation") -> (w472:T15)
            n178 = Bundle By Name(cluster=w474, "Configuration.Measurement.W-Sweep"=w472) -> (w473:T16)
          }
        }
        n179 = call <vilib>:"Add State(s) to Queue__jki_lib_state_machine.vi"("State(s) in (\"\")"=w433) -> ("States Out"=w432:string)  [unwired: 14 in]
      }
      frame "Configuration: Create Main" {
        n180 = case shown="\"Free\", Default" w486 {
          tunnel: w485 -> [w491 w499 w511 w518]
          tunnel: [w490 w500 w510 w519] -> w484
          frame "Free", Default {
            w498 = T18 {"Measurement.Type"=enum."Free", "Hardware"={"SMU"={"Enable"=FALSE, "SMU Model"="", "Configuration"={"VISA Resource"="", "Channel"=""}}, "LIA"={"Enable"=FALSE, "LIA Model"="", "Configuration"={"VISA Resource"=""}}, "OPM"={"Enable"=FALSE, "OPM Model"="", "Configuration"={"VISA Resource"=""}}, "OPA"={"Enable"=FALSE, "OPA Model"="", "Configuration"={"Serial Number"=""}}}}  # Configuration
            n181 = Unbundle By Name(w491) -> ("Configuration.SMU"=w496:T7, "Configuration.LIA"=w495:T9, "Configuration.OPM"=w494:T11, "Configuration.OPA"=w493:T13)
            n182 = Bundle By Name(cluster=w498, "Measurement.Type"=Measurement.Type--Enum."Free", "Hardware.SMU"=w496, "Hardware.LIA"=w495, "Hardware.OPM"=w494, "Hardware.OPA"=w493) -> (w492:T18)
            n183 = Bundle By Name(cluster=w491, "Configuration"=w492) -> (w490:T16)
          }
          frame "I-V Curve" {
            w507 = T18 {"Measurement.Type"=enum."Free", "Hardware"={"SMU"={"Enable"=FALSE, "SMU Model"="", "Configuration"={"VISA Resource"="", "Channel"=""}}, "LIA"={"Enable"=FALSE, "LIA Model"="", "Configuration"={"VISA Resource"=""}}, "OPM"={"Enable"=FALSE, "OPM Model"="", "Configuration"={"VISA Resource"=""}}, "OPA"={"Enable"=FALSE, "OPA Model"="", "Configuration"={"Serial Number"=""}}}}  # Configuration
            n184 = Unbundle By Name(w499) -> ("Configuration.SMU"=w505:T7, "Configuration.LIA"=w504:T9, "Configuration.OPM"=w503:T11, "Configuration.OPA"=w502:T13)
            n185 = Bundle By Name(cluster=w507, "Measurement.Type"=Measurement.Type--Enum."Free", "Hardware.SMU"=w505, "Hardware.LIA"=w504, "Hardware.OPM"=w503, "Hardware.OPA"=w502) -> (w501:T18)
            n186 = Bundle By Name(cluster=w499, "Configuration"=w501) -> (w500:T16)
          }
          frame "Wavelength sweeping" {
            w517 = T20 {"Measurement.Type"=enum."Free", "Hardware"={"SMU"={"Enable"=FALSE, "SMU Model"="", "Configuration"={"VISA Resource"="", "Channel"=""}}, "LIA"={"Enable"=FALSE, "LIA Model"="", "Configuration"={"VISA Resource"=""}}, "OPM"={"Enable"=FALSE, "OPM Model"="", "Configuration"={"VISA Resource"=""}}, "OPA"={"Enable"=FALSE, "OPA Model"="", "Configuration"={"Serial Number"=""}}}, "Measurement"={"SMU Voltage, V"=0.0, "OPA Start wavelength, nm"=0.0, "OPA Stop wavelength, nm"=0.0, "OPA Scan resolution, nm"=0.0, "OPA Number or points"=0, "Integration time, sec"=0.0, "Delay time, ms"=0, "Accumulation"=0}}  # Configuration
            n187 = Unbundle By Name(w511) -> ("Configuration.SMU"=w516:T7, "Configuration.LIA"=w515:T9, "Configuration.OPM"=w514:T11, "Configuration.OPA"=w513:T13, "Configuration.Measurement.W-Sweep"=w512:T15)
            n188 = Bundle By Name(cluster=w517, "Measurement.Type"=Measurement.Type--Enum."Wavelength sweeping", "Hardware.SMU"=w516, "Hardware.LIA"=w515, "Hardware.OPM"=w514, "Hardware.OPA"=w513, "Measurement"=w512) -> (w509:T20)
            n189 = Bundle By Name(cluster=w511, "Configuration"=w509) -> (w510:T16)
          }
          frame "Photocurrent mapping" {
            w526 = T18 {"Measurement.Type"=enum."Free", "Hardware"={"SMU"={"Enable"=FALSE, "SMU Model"="", "Configuration"={"VISA Resource"="", "Channel"=""}}, "LIA"={"Enable"=FALSE, "LIA Model"="", "Configuration"={"VISA Resource"=""}}, "OPM"={"Enable"=FALSE, "OPM Model"="", "Configuration"={"VISA Resource"=""}}, "OPA"={"Enable"=FALSE, "OPA Model"="", "Configuration"={"Serial Number"=""}}}}  # Configuration
            n190 = Unbundle By Name(w518) -> ("Configuration.SMU"=w524:T7, "Configuration.LIA"=w523:T9, "Configuration.OPM"=w522:T11, "Configuration.OPA"=w521:T13)
            n191 = Bundle By Name(cluster=w526, "Measurement.Type"=Measurement.Type--Enum."Free", "Hardware.SMU"=w524, "Hardware.LIA"=w523, "Hardware.OPM"=w522, "Hardware.OPA"=w521) -> (w520:T18)
            n192 = Bundle By Name(cluster=w518, "Configuration"=w520) -> (w519:T16)
          }
        }
        n193 = call <vilib>:"Add State(s) to Queue__jki_lib_state_machine.vi"("State(s) in (\"\")"=w489) -> ("States Out"=w488:string)  [unwired: 14 in]
      }
    }
  }
